vi "Parallel Mode Read.vi"(8 "error in":errorcluster, 11 "Parallel Mode in":refnum<class "Parallel Mode.lvclass">) -> (0 "error out":errorcluster, 1 "Changed or First Call?":bool, 2 "Parallel Mode ACT":bool, 3 "Parallel Mode out":refnum<class "Parallel Mode.lvclass">)   [LabVIEW 2023, in "Parallel Mode.lvclass"]
uses:
  Parallel Mode.lvclass
  Parallel Mode.lvclass/Parallel Mode.ctl
  c55f003c-d6ba-43b5-974c-5d851376f510.vi
  <vilib>/ADAS Replay HIL/Channels/Tag Wrapper/Tag Wrapper.lvlib
  <vilib>/ADAS Replay HIL/Channels/Tag Wrapper/Polymorphic/Read Channel (Boolean).vi
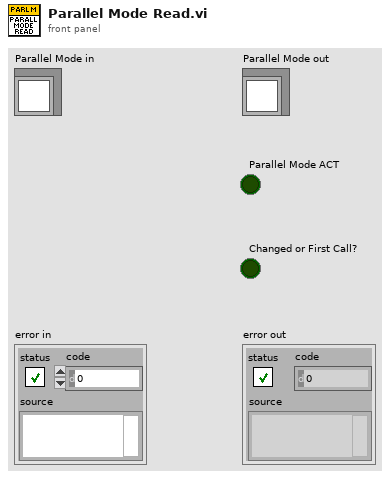
[diagram p1: front panel]
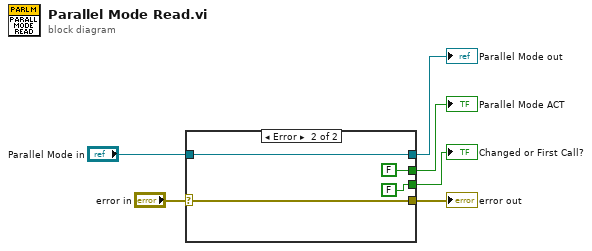
[diagram p0: block diagram]
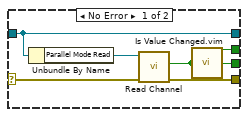
[diagram p2: hidden frame]
diagram:
  n1 = case shown="Error" "error in" {
    selector: "error in" -> [w7 w16]
    tunnel: [w8 w16] -> w5
    tunnel: [w11 w15] -> w3
    tunnel: "Parallel Mode in" -> [w11 w15]
    tunnel: [w10 FALSE ("Value out")] -> w2
    tunnel: [w9 FALSE ("changed or first call?")] -> w1
    frame No Error {
      n2 = Unbundle By Name(w11) -> ("Parallel Mode Read"=w12:refnum<k21>)
      n3 = call-poly <vilib>:"Read Channel.vi"("error in"=w7, "ADAS HIL Channel in"=w12) -> ("error out"=w8:errorcluster, "Value out"=w10:bool)  [unwired: 6 in, 2 out]
      n4 = call "Is Value Changed.vim"("value"=w10) -> ("changed or first call?"=w9:bool)
    }
    frame Error {
    }
  }
  "error out" <- w5
  "Parallel Mode out" <- w3
  "Parallel Mode ACT" <- w2
  "Changed or First Call?" <- w1
